vi "get_config_cluster.vi"(8 "error in (no error)":errorcluster, 11 "GenericPlugin in":refnum<class "InstrumentDL090324.lvclass">) -> (0 "error out":errorcluster, 2 "config cluster (variant)":variant, 3 "GenericPlugin out":refnum<class "InstrumentDL090324.lvclass">)   [LabVIEW 2010, in "InstrumentDL090324.lvclass"]
uses:
  InstrumentDL090324.lvclass
  InstrumentDL090324.lvclass/InstrumentDL090324.ctl
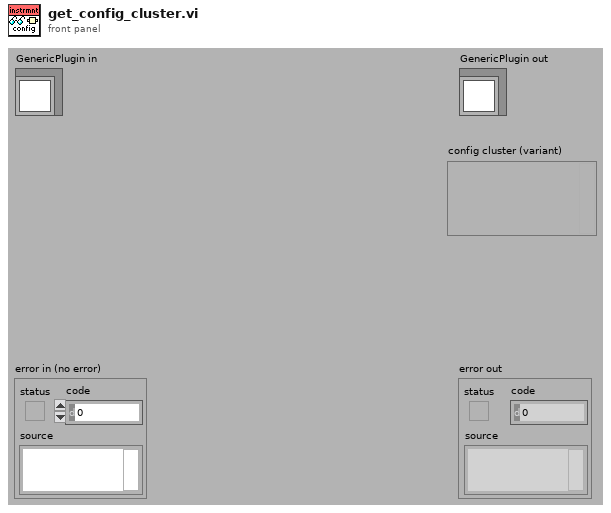
[diagram p1: front panel]
types:
  T1 = typedef "InstrumentDL090324.lvclass/config_data_cluster.ctl" = cluster{"detectors":T2[], "LSID":T3, "light source":T2[]}
  T2 = typedef "plugin_specification.ctl" = cluster{"class path":string, "configuration":string, "label":string, "settings name":string}
  T3 = typedef "LSID_cluster.ctl" = cluster{"identifier":string, "revision":i32}
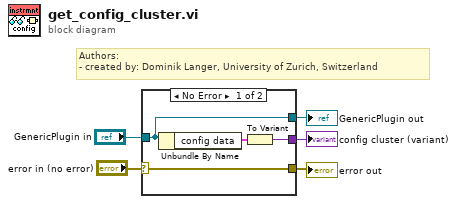
[diagram p0: block diagram]
diagram:
  # "Authors: \n- created by: Dominik Langer, University of Zurich, Switzerland"
  n1 = case shown="No Error" "error in (no error)" {
    selector: "error in (no error)" -> [w6 w11]
    tunnel: "GenericPlugin in" -> [w8 w10]
    tunnel: [w8 w10] -> w2
    tunnel: [w7 _] -> w3
    tunnel: [w6 w11] -> w1
    frame No Error {
      n2 = Unbundle By Name(w8) -> ("config data"=w9:T1)
      n3 = To Variant(anything=w9) -> (Variant=w7:variant)
    }
    frame Error {
    }
  }
  "error out" <- w1
  "GenericPlugin out" <- w2
  "config cluster (variant)" <- w3
